vi "ModifyGraph Log.vi"(8 "error in (no error)":errorcluster, 10 "Label":cluster{"bottom":T1, "left":T1}, 11 "ITX Commands in":refnum<class "ITX Commands.lvclass">) -> (0 "error out":errorcluster, 3 "ITX Commands out":refnum<class "ITX Commands.lvclass">)   [LabVIEW 2020, in "ITX Commands.lvclass"]
uses:
  ITX Commands.lvclass
  typedefs/log--enum.ctl
panel:
  out "resulting string":string
  # "n=0: normal axis\nn=1: log base 10\nn=2: log base 2"
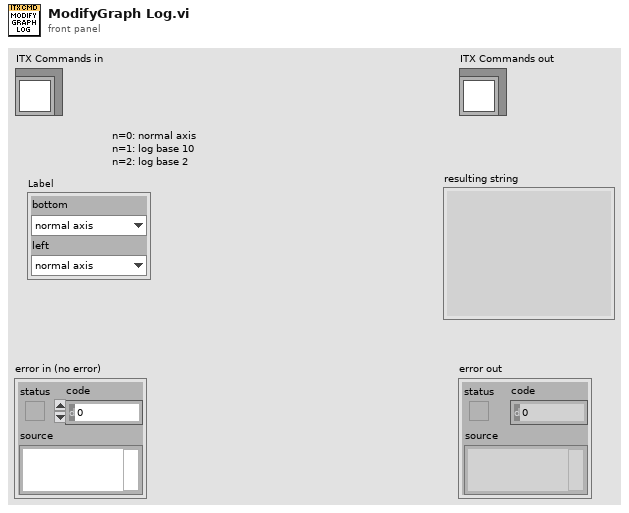
[diagram p1: front panel]
types:
  T1 = typedef "ITX Commands.lvclass/log--enum.ctl" = enum16{"normal axis", "log base 10", "log base 2"}
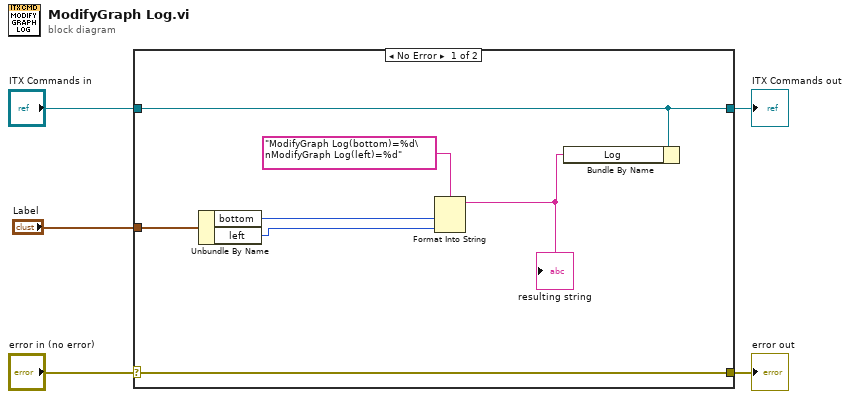
[diagram p0: block diagram]
diagram:
  n1 = case shown="No Error" "error in (no error)" {
    selector: "error in (no error)" -> [w12 w14]
    tunnel: [w12 w14] -> w4
    tunnel: [w10 w13] -> w2
    tunnel: "ITX Commands in" -> [w10 w13]
    tunnel: "Label" -> [w8 _]
    frame No Error {
      n2 = Unbundle By Name(w8) -> ("bottom"=w7:T1, "left"=w6:T1)
      n3 = Format Into String(format string="ModifyGraph Log(bottom)=%d\nModifyGraph Log(left)=%d", w7, w6) -> (resulting string=w9:string)  [unwired: 2 in, 1 out]
      "resulting string" <- w9
      n4 = Bundle By Name(cluster=w10, "Log"=w9) -> ()  [unwired: 1 out]
    }
    frame Error {
    }
  }
  "error out" <- w4
  "ITX Commands out" <- w2
